vi "FLIP_FLOP.vi"() -> ()   [LabVIEW 2019]
panel:
  in  "OK Button":bool
  in  "stop":bool
  out ".not. (x .xor. y)?":bool
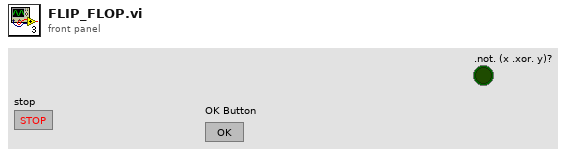
[diagram p1: front panel]
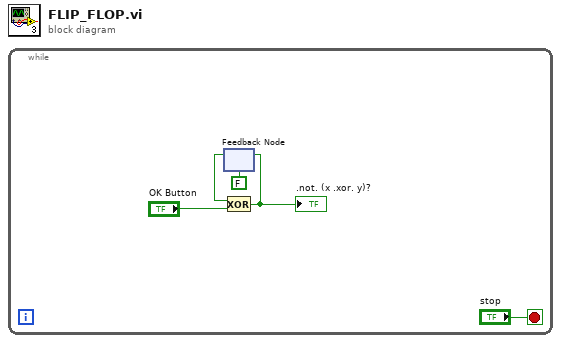
[diagram p0: block diagram]
diagram:
  n1 = while {
    stop <- "stop" stop-if-true
    n2 = feedback #1(FALSE) -> (w4:bool)
    n3 = Exclusive Or(1:"OK Button", 2:w4) -> (0:w3:bool)
    ".not. (x .xor. y)?" <- w3
    n4 = feedback-in #1(w3) -> ()
  }
